vi "Login1.vi"() -> ()   [LabVIEW 2013]
uses:
  <vilib>/addons/database/Connection.llb/DB Tools Open Connec (String).vi
  FYP_LabviewGlobal(SubVI).vi
  <vilib>/addons/database/NI_Database_API.lvlib
panel:
  in  "Quit":bool
  in  "LogInAsAdmin":bool
  in  "SignUp":bool
  in  "Login":bool
  in  "Password":string
  in  "Admin no":string
  # "Welcome to \nIntelligent Assessment & Advisory\nE-learning System"
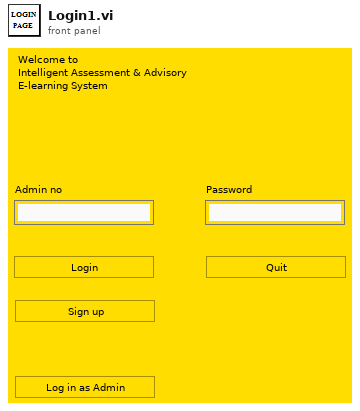
[diagram p1: front panel]
types:
  T1 = enum8{"Enabled", "Disabled", "Disabled and Grayed Out"}
  T2 = typedef "NI_Database_API.lvlib/Conn ObjectReference.ctl" = refnum<k1>
  T3 = enum32{"Invalid", "Standard", "Closed", "Hidden", "Minimized", "Maximized"}
  T4 = cluster{"Admin no":string, "date/time string":string, string}
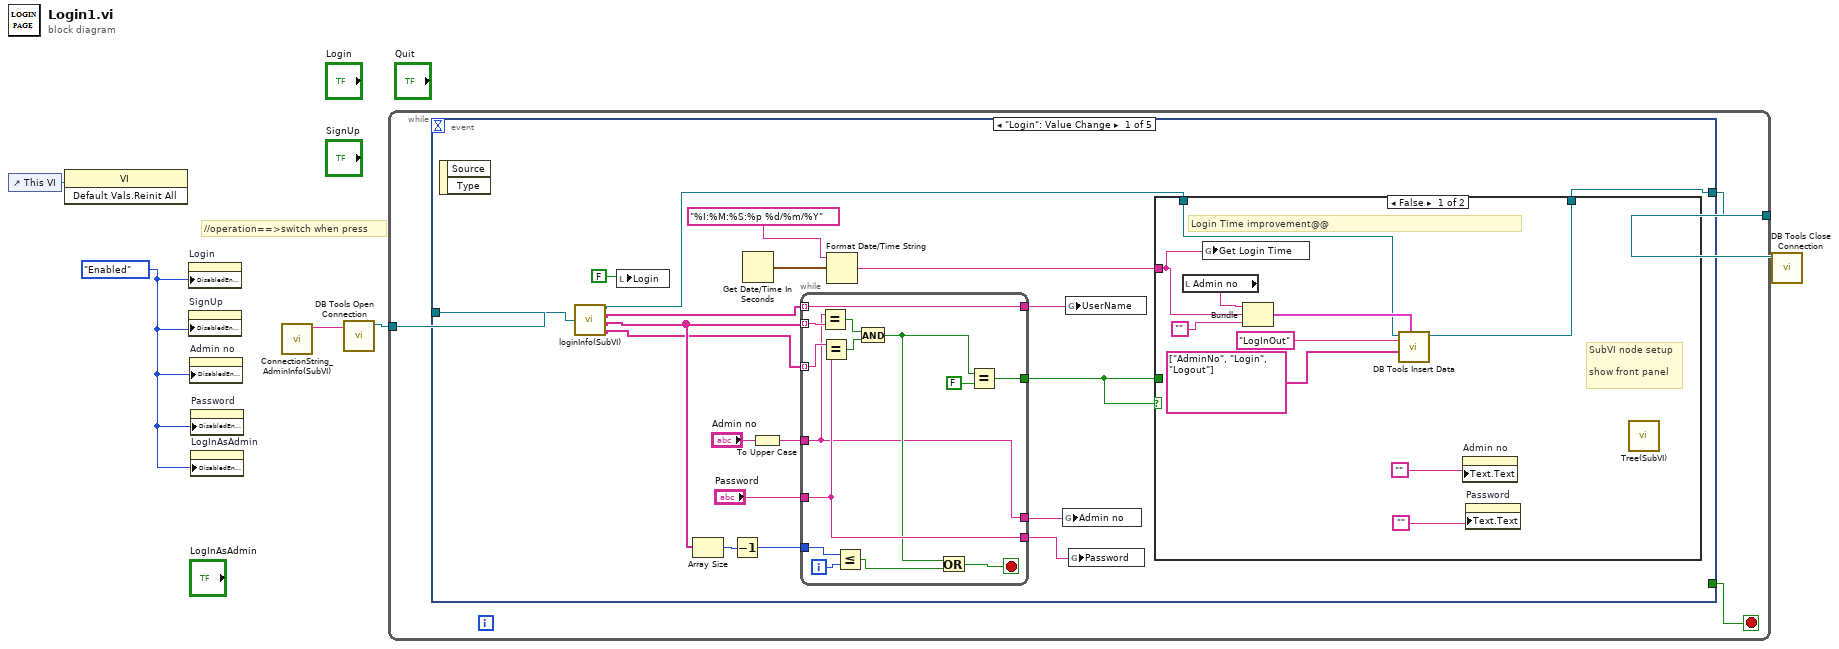
[diagram p0: block diagram]
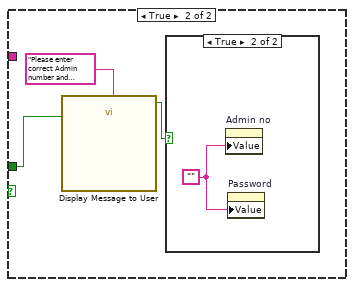
[diagram p2: hidden frame]
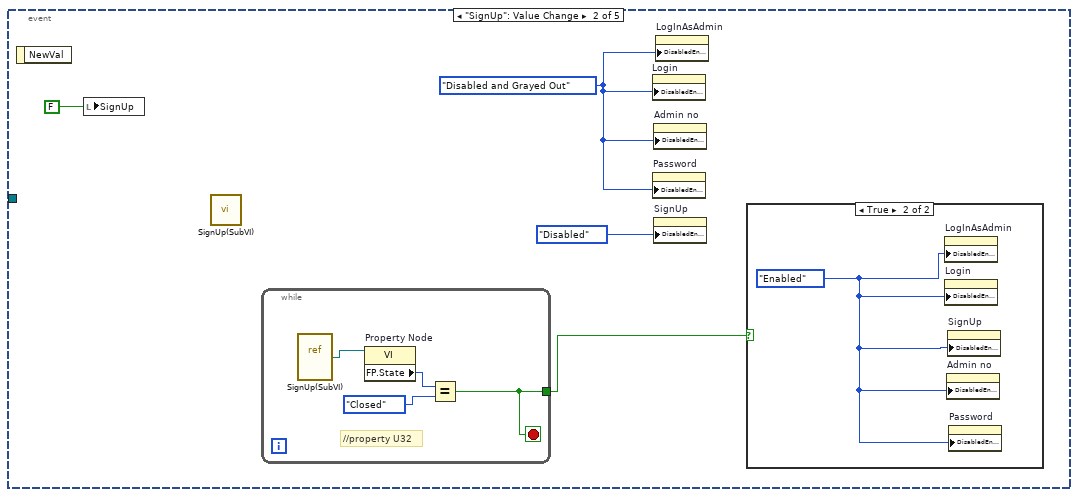
[diagram p4: hidden frame]
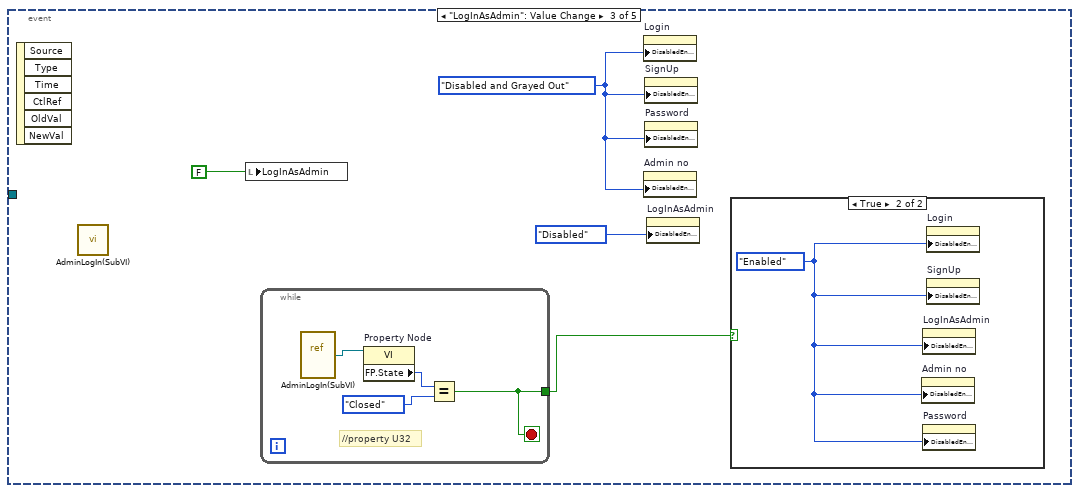
[diagram p6: hidden frame]
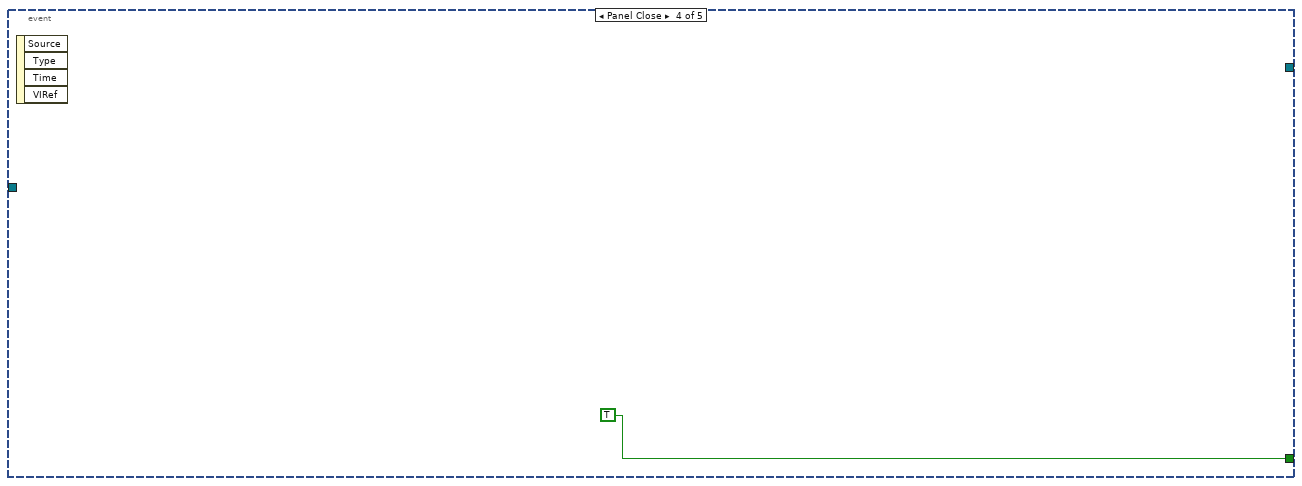
[diagram p8: hidden frame]
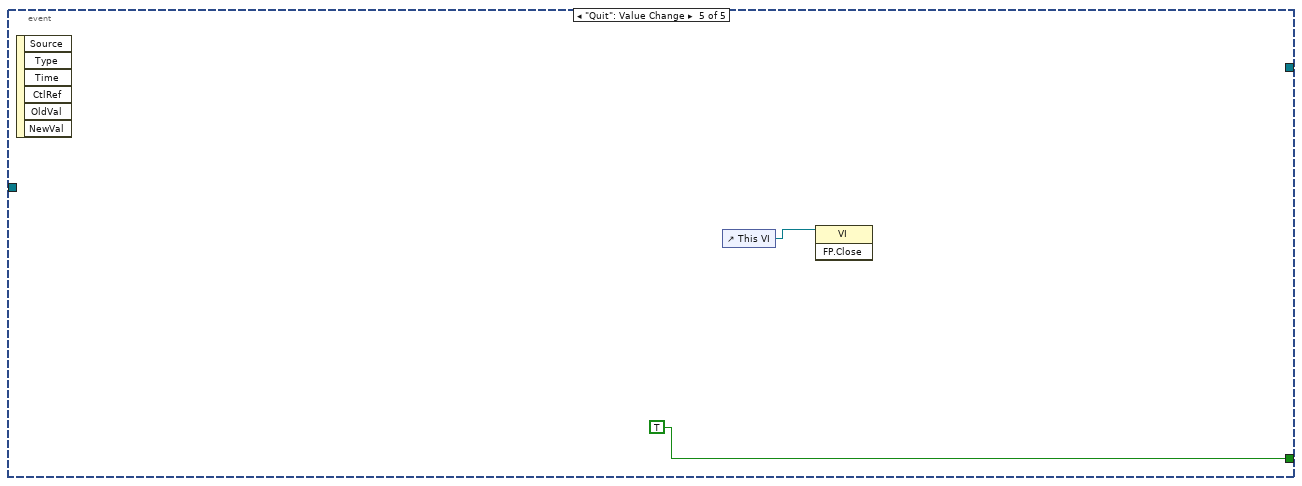
[diagram p9: hidden frame]
diagram:
  w1 = T1."Enabled"
  # "//operation==>switch when press"
  n1 = control-ref of="This VI"() -> (w5:refnum<vi>)
  n2 = invoke class="VI" method="Default Vals.Reinit All"(reference=w5) -> ()  [unwired: 2 in, 3 out]
  n3 = property on="Login" class="Bool (strict)"("DisabledEnum"=w1) -> ()  [unwired: 2 in, 2 out]
  n4 = property on="SignUp" class="Bool (strict)"("DisabledEnum"=w1) -> ()  [unwired: 2 in, 2 out]
  n5 = property on="Admin no" class="Str"("DisabledEnum"=w1) -> ()  [unwired: 2 in, 2 out]
  n6 = property on="Password" class="Str"("DisabledEnum"=w1) -> ()  [unwired: 2 in, 2 out]
  n7 = property on="LogInAsAdmin" class="Bool (strict)"("DisabledEnum"=w1) -> ()  [unwired: 2 in, 2 out]
  n8 = call "ConnectionString_AdminInfo(SubVI).vi"() -> ("ConnectionString"=w2:string)  [unwired: 11 in]
  n9 = call-poly <vilib>:"DB Tools Open Connection.vi"("connection information"=w2) -> ("connection reference"=w3:T2)  [unwired: 7 in, 1 out]
  n10 = while {
    tunnel: [w8] -> w4
    tunnel: w3 -> [w7]
    stop <- w6 stop-if-true
    n11 = event shown="[0] \"Login\": Value Change" {
      selector: _ -> [_ _ _ _ _]
      dyn-events: _ -> [_ _ _ _ _]
      timeout: _ -> [_ _ _ _ _]
      tunnel: [w9 _ _ _ _] -> w8
      tunnel: w7 -> [w14 _ _ _ _]
      tunnel: [_ _ _ TRUE TRUE] -> w6
      event "Login": Value Change {
        n12 = event-data() -> ()  [unwired: 1 in, 2 out]
        n13 = call "loginInfo(SubVI).vi"("connection reference 2"=w14) -> ("connection reference 4"=w10:T2, "GetUserName 3"=w13:string[], "GetAdminNo 3"=w12:string[], "GetPassword 3"=w11:string[])
        n14 = local write "Login"(FALSE) -> ()
        n15 = Array Size(array=w12) -> (size(s)=w25:i32)
        n16 = Decrement(x=w25) -> (x-1=w24:i32)
        n17 = Get Date/Time In Seconds() -> (seconds since 1Jan1904=w18:timestamp)
        n18 = To Upper Case(1:"Admin no") -> (0:w23:string)
        n19 = while {
          tunnel: w24 -> [w55]
          tunnel: [w51] -> w21
          tunnel: w13 -> [w51] mode=indexing
          tunnel: w12 -> [w50] mode=indexing
          tunnel: w11 -> [w47] mode=indexing
          tunnel: w23 -> [w42]
          tunnel: "Password" -> [w45]
          tunnel: [w45] -> w20
          tunnel: [w42] -> w19
          tunnel: [w44] -> w17
          i -> [w54]
          stop <- w52 stop-if-true
          n20 = Equal?(x=w42, y=w50) -> (x = y?=w49:bool)
          n21 = Equal?(x=w47, y=w45) -> (x = y?=w48:bool)
          n22 = Less Or Equal?(x=w55, y=w54) -> (x <= y?=w53:bool)
          n23 = And(x=w49, y=w48) -> (x .and. y?=w43:bool)
          n24 = Or(x=w43, y=w53) -> (x .or. y?=w52:bool)
          n25 = Equal?(x=w43, y=FALSE) -> (x = y?=w44:bool)
        }
        n26 = Format Date/Time String(time format string (%c)="%I:%M:%S:%p %d/%m/%Y", seconds (now)=w18) -> (date/time string=w16:string)  [unwired: 1 in]
        n27 = global write "FYP_LabviewGlobal(SubVI).vi" "Admin no"(w19) -> ()
        n28 = global write "FYP_LabviewGlobal(SubVI).vi" "UserName"(w21) -> ()
        n29 = global write "FYP_LabviewGlobal(SubVI).vi" "Password"(w20) -> ()
        n30 = case shown="False" w17 {
          tunnel: w17 -> [_ w38]
          tunnel: w16 -> [w37 _]
          tunnel: w10 -> [w34 _]
          tunnel: [w31 _] -> w9
          frame False {
            # "Login Time improvement@@"
            # "SubVI node setup\n\nshow front panel"
            n31 = local read "Admin no"() -> (w30:string)
            n32 = global write "FYP_LabviewGlobal(SubVI).vi" "Get Login Time"(w37) -> ()
            n33 = Bundle("Admin no"=w30, "date/time string"=w37, "") -> (w35:T4)  [unwired: 1 in]
            n34 = call <vilib>:"DB Tools Insert Data.vi"("data"=w35, "columns"=string[] ["AdminNo", "Login", "Logout"], "table"="LogInOut", "connection reference"=w34) -> ("connection reference out"=w31:T2)  [unwired: 6 in, 1 out]
            n35 = property on="Admin no" class="Str"("Text.Text"="") -> ()  [unwired: 2 in, 2 out]
            n36 = property on="Password" class="Str"("Text.Text"="") -> ()  [unwired: 2 in, 2 out]
            n37 = call "Tree(SubVI).vi"() -> ()  [unwired: 12 in]
          }
          frame True {
            n38 = call "Display Message to User"("Enable"=w38, "Message"="Please enter correct Admin number and Password") -> ("OK"=w39:bool)  [unwired: 8 in, 1 out]
            n39 = case shown="True" w39 {
              frame False {
              }
              frame True {
                w41 = ""
                n40 = property on="Admin no" class="Str"("Value"=w41) -> ()  [unwired: 2 in, 2 out]
                n41 = property on="Password" class="Str"("Value"=w41) -> ()  [unwired: 2 in, 2 out]
              }
            }
          }
        }
      }
      event "SignUp": Value Change {
        w56 = T1."Disabled and Grayed Out"
        n42 = event-data() -> ()  [unwired: 1 in, 1 out]
        n43 = local write "SignUp"(FALSE) -> ()
        n44 = call "SignUp(SubVI).vi"() -> ()  [unwired: 12 in]
        n45 = while {
          tunnel: [w62] -> w59
          stop <- w62 stop-if-true
          # "//property U32"
          n46 = vi-ref "SignUp(SubVI).vi"() -> (w64:refnum<vi>)
          n47 = property on="Property Node" class="VI"(reference=w64) -> ("FP.State"=w63:T3)  [unwired: 1 in, 2 out]
          n48 = Equal?(x=w63, y=T3."Closed") -> (x = y?=w62:bool)
        }
        n49 = property on="Login" class="Bool (strict)"("DisabledEnum"=w56) -> ()  [unwired: 2 in, 2 out]
        n50 = property on="Password" class="Str"("DisabledEnum"=w56) -> ()  [unwired: 2 in, 2 out]
        n51 = property on="Admin no" class="Str"("DisabledEnum"=w56) -> ()  [unwired: 2 in, 2 out]
        n52 = property on="SignUp" class="Bool (strict)"("DisabledEnum"=T1."Disabled") -> ()  [unwired: 2 in, 2 out]
        n53 = property on="LogInAsAdmin" class="Bool (strict)"("DisabledEnum"=w56) -> ()  [unwired: 2 in, 2 out]
        n54 = case shown="True" w59 {
          frame False {
          }
          frame True {
            w60 = T1."Enabled"
            n55 = property on="LogInAsAdmin" class="Bool (strict)"("DisabledEnum"=w60) -> ()  [unwired: 2 in, 2 out]
            n56 = property on="Login" class="Bool (strict)"("DisabledEnum"=w60) -> ()  [unwired: 2 in, 2 out]
            n57 = property on="Admin no" class="Str"("DisabledEnum"=w60) -> ()  [unwired: 2 in, 2 out]
            n58 = property on="SignUp" class="Bool (strict)"("DisabledEnum"=w60) -> ()  [unwired: 2 in, 2 out]
            n59 = property on="Password" class="Str"("DisabledEnum"=w60) -> ()  [unwired: 2 in, 2 out]
          }
        }
      }
      event "LogInAsAdmin": Value Change {
        w66 = T1."Disabled and Grayed Out"
        n60 = event-data() -> ()  [unwired: 1 in, 6 out]
        n61 = call "AdminLogIn(SubVI).vi"() -> ()  [unwired: 12 in]
        n62 = local write "LogInAsAdmin"(FALSE) -> ()
        n63 = while {
          tunnel: [w72] -> w65
          stop <- w72 stop-if-true
          # "//property U32"
          n64 = vi-ref "AdminLogIn(SubVI).vi"() -> (w70:refnum<vi>)
          n65 = property on="Property Node" class="VI"(reference=w70) -> ("FP.State"=w73:T3)  [unwired: 1 in, 2 out]
          n66 = Equal?(x=w73, y=T3."Closed") -> (x = y?=w72:bool)
        }
        n67 = property on="Login" class="Bool (strict)"("DisabledEnum"=w66) -> ()  [unwired: 2 in, 2 out]
        n68 = property on="Admin no" class="Str"("DisabledEnum"=w66) -> ()  [unwired: 2 in, 2 out]
        n69 = property on="SignUp" class="Bool (strict)"("DisabledEnum"=w66) -> ()  [unwired: 2 in, 2 out]
        n70 = property on="Password" class="Str"("DisabledEnum"=w66) -> ()  [unwired: 2 in, 2 out]
        n71 = property on="LogInAsAdmin" class="Bool (strict)"("DisabledEnum"=T1."Disabled") -> ()  [unwired: 2 in, 2 out]
        n72 = case shown="True" w65 {
          frame False {
          }
          frame True {
            w69 = T1."Enabled"
            n73 = property on="Admin no" class="Str"("DisabledEnum"=w69) -> ()  [unwired: 2 in, 2 out]
            n74 = property on="LogInAsAdmin" class="Bool (strict)"("DisabledEnum"=w69) -> ()  [unwired: 2 in, 2 out]
            n75 = property on="Password" class="Str"("DisabledEnum"=w69) -> ()  [unwired: 2 in, 2 out]
            n76 = property on="Login" class="Bool (strict)"("DisabledEnum"=w69) -> ()  [unwired: 2 in, 2 out]
            n77 = property on="SignUp" class="Bool (strict)"("DisabledEnum"=w69) -> ()  [unwired: 2 in, 2 out]
          }
        }
      }
      event Panel Close {
        n78 = event-data() -> ()  [unwired: 1 in, 4 out]
      }
      event "Quit": Value Change {
        n79 = event-data() -> ()  [unwired: 1 in, 6 out]
        n80 = control-ref of="This VI"() -> (w75:refnum<vi>)
        n81 = invoke class="VI" method="FP.Close"(reference=w75) -> ()  [unwired: 2 in, 3 out]
      }
    }
  }
  n82 = call <vilib>:"DB Tools Close Connection.vi"("connection reference"=w4) -> ()  [unwired: 6 in, 1 out]
